vi "DAC (B).vi"(8 "error in (no error)":errorcluster, 11 "Dac":refnum<k24>) -> (0 "error out":errorcluster)   [LabVIEW 2011]
doc: "Control the digital/analog converter with constant values(basic version)."
uses:
  C:/Program Files/Metrohm Autolab/Autolab SDK 1.10/EcoChemie.Autolab.Sdk.dll
  EcoChemie.Autolab.Sdk.dll
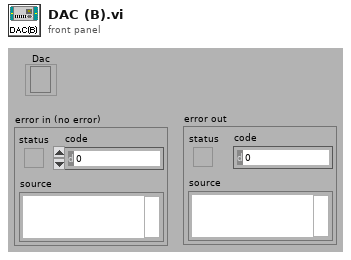
[diagram p1: front panel]
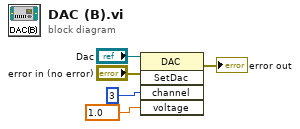
[diagram p0: block diagram]
diagram:
  n1 = invoke class="DAC" method="SetDac"(reference="Dac", error in="error in (no error)", "channel"=3, "voltage"=1.0) -> (error out=→"error out":errorcluster)  [unwired: 1 in, 4 out]
